vi "Receive PS Dataset.vi"(8 "error in (no error)":errorcluster, 10 "PS Dataset":cluster{"Connected":bool, "Data":dbl[]}, 11 "Test in":refnum<class "Test.lvclass">) -> (0 "error out":errorcluster, 3 "Test out":refnum<class "Test.lvclass">)   [LabVIEW 2019, in "Test.lvlib" / "Test.lvclass"]
uses:
  Test.lvclass
  Test.lvclass/Test.ctl
  Platform/Platform Messages/Get Instrument Dataset Msg/Get Instrument Data Msg.lvclass/Get Instrument Data Msg.ctl
  <vilib>/ActorFramework/Message Enqueuer/Message Enqueuer.lvclass/Message Enqueuer.ctl
  <vilib>/ActorFramework/Message Enqueuer/Enqueue.vi
  Platform/Platform Messages/Get Instrument Dataset Msg/Get Instrument Data Msg.lvclass
  C:/Program Files (x86)/National Instruments/LabVIEW 2019/vi.lib/ActorFramework/Message/Message.lvclass
  <vilib>/ActorFramework/Message Priority Queue/Priority Enqueue.vi
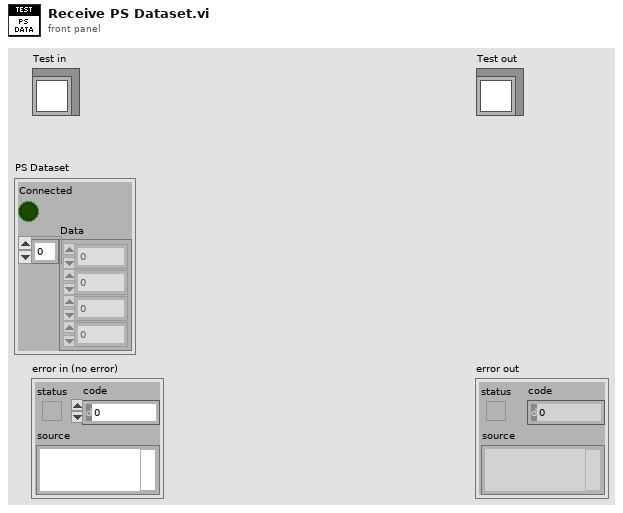
[diagram p1: front panel]
types:
  T1 = map{string, cluster{"Selected Heads":string, "Instrument":refnum<class "Message Enqueuer.lvclass">, "Platform":refnum<class "Message Enqueuer.lvclass">}}
  T2 = typedef "Test.lvlib/Cobra Data.ctl" = cluster{"M2 Dataset":cluster{"Read Temp":dbl, "Feedback":u8, "Set Temp":dbl}, "M1 Dataset":cluster{"Read Temp":dbl, "Feedback":u8, "Set Temp":dbl}, "Comp":bool}
  T3 = cluster{"Selected Heads":string, "Instrument":refnum<class "Message Enqueuer.lvclass">, "Platform":refnum<class "Message Enqueuer.lvclass">}
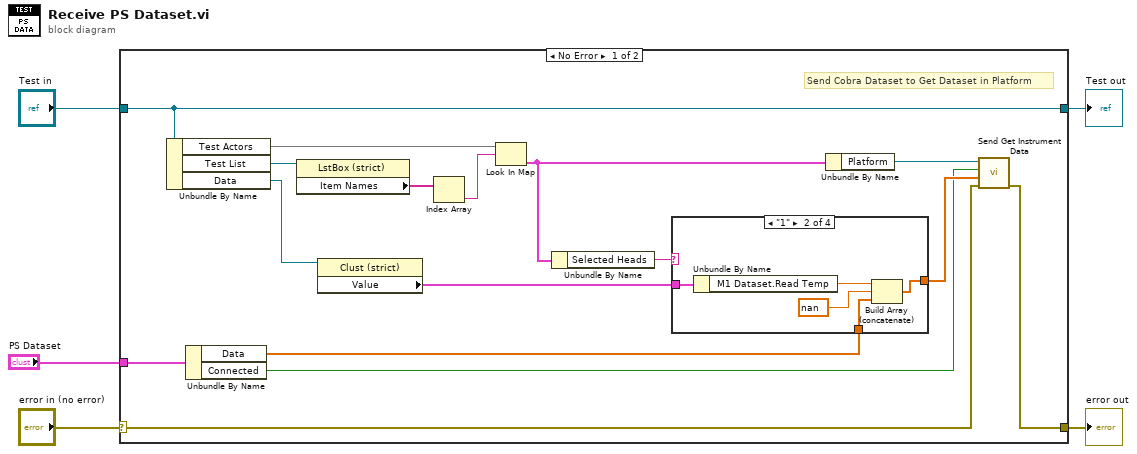
[diagram p0: block diagram]
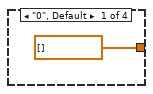
[diagram p2: hidden frame]
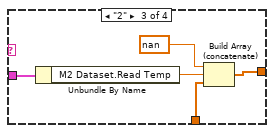
[diagram p3: hidden frame]
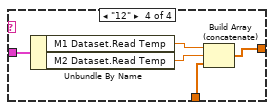
[diagram p4: hidden frame]
diagram:
  n1 = case shown="No Error" "error in (no error)" {
    selector: "error in (no error)" -> [w21 w39]
    tunnel: [w20 w39] -> w4
    tunnel: [w17 w38] -> w2
    tunnel: "Test in" -> [w17 w38]
    tunnel: "PS Dataset" -> [w13 _]
    frame No Error {
      # "Send Cobra Dataset to Get Dataset in Platform"
      n2 = Unbundle By Name(w17) -> ("Test Actors"=w16:T1, "Test List"=w18:refnum<vi>, "Data"=w10:refnum<vi>)
      n3 = Unbundle By Name(w13) -> ("Data"=w8:dbl[], "Connected"=w9:bool)
      n4 = property class="LstBox (strict)"(reference=w18) -> ("Item Names"=w19:string[])  [unwired: 1 in, 2 out]
      n5 = property class="Clust (strict)"(reference=w10) -> ("Value"=w12:T2)  [unwired: 1 in, 2 out]
      n6 = Index Array(array=w19) -> (element=w15:string)  [unwired: 1 in]
      n7 = Look In Map(map=w16, key=w15) -> (value=w7:T3)  [unwired: 1 in, 1 out]
      n8 = Unbundle By Name(w7) -> ("Selected Heads"=w6:string)
      n9 = case shown="\"1\"" w6 {
        tunnel: w8 -> [_ w24 w28 w35]
        tunnel: w12 -> [_ w27 w32 w37]
        tunnel: [dbl[] [] w25 w30 w34] -> w11
        frame "0", Default {
        }
        frame "1" {
          n10 = Unbundle By Name(w27) -> ("M1 Dataset.Read Temp"=w26:dbl)
          n11 = Build Array (concatenate)(w26, nan, w24) -> (w25:dbl[])
        }
        frame "2" {
          n12 = Unbundle By Name(w32) -> ("M2 Dataset.Read Temp"=w31:dbl)
          n13 = Build Array (concatenate)(nan, w31, w28) -> (w30:dbl[])
        }
        frame "12" {
          n14 = Unbundle By Name(w37) -> ("M1 Dataset.Read Temp"=w33:dbl, "M2 Dataset.Read Temp"=w36:dbl)
          n15 = Build Array (concatenate)(w33, w36, w35) -> (w34:dbl[])
        }
      }
      n16 = Unbundle By Name(w7) -> ("Platform"=w14:refnum<class "Message Enqueuer.lvclass">)
      n17 = call "Send Get Instrument Data.vi"("error in (no error)"=w21, "Data"=w11, "Connection"=w9, "Message Enqueuer"=w14) -> ("error out"=w20:errorcluster)  [unwired: 6 in, 1 out]
    }
    frame Error {
    }
  }
  "error out" <- w4
  "Test out" <- w2
